vi "Log Add Msg.vi"(1 "Result":string, 2 "Communication":string, 3 "Description":string) -> (0 "Out Msg":string)   [LabVIEW 2018]
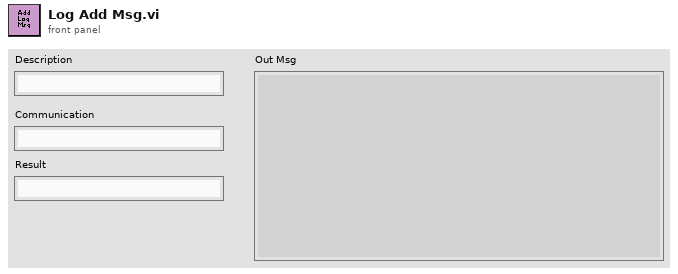
[diagram p1: front panel]
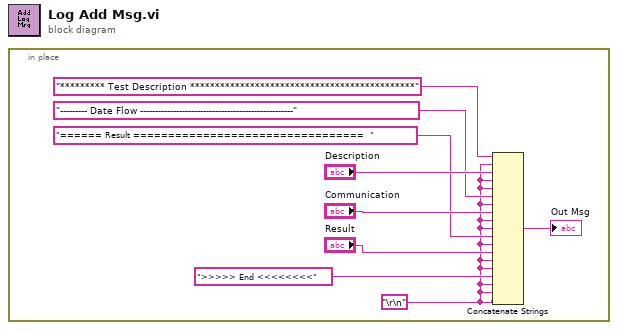
[diagram p0: block diagram]
diagram:
  n1 = in-place {
    w1 = "\r\n"
    n2 = Concatenate Strings("********* Test Description *********************************************", w1, "Description", w1, w1, "--------- Date Flow ---------------------------------------------------", w1, "Communication", w1, w1, "====== Result =================================  ", w1, "Result", w1, w1, ">>>>> End <<<<<<<<", w1, w1, w1) -> (→"Out Msg":string)
  }
